vi "CALC_PAR_SEL.vi"(0 "VISA IN":refnum<visa-resource-name>, 1 "Measurement":string="CH1_S11_1", 5 "error in":errorcluster, 7 "Channel":i32=1) -> (14 "VISA Out":refnum<visa-resource-name>, 19 "error out":errorcluster)   [LabVIEW 2018, in "PNA-X.lvlib"]
doc: "CALCulate<cnum>:PARameter:SELect <Mname> \n1559\n\n(Read-Write) Sets the selected measurement. Most CALC: commands require that this command be \nsent before a setting change is made. One measurement on each channel can be selected at the same \ntime. To obtain a list of currently named measurements, use CALC:PAR:CAT? \nParameters \n<cnum> Channel number of the measurement to be selected. If unspecified, <cnum> is \nset to 1. \n<Mname> String - Name of the measurement. (Do NOT include the parameter name.) \nExamples CALC:PAR:SEL 'TEST' \ncalculate2:parameter:select 'test' \nQuery Syntax CALCulate:PARameter:SELect? \nReturn Type String \nDefault The preset measurement name is \"CH1_S11_1\" \nLast modified: \nApril 19, 2007 MX Added ADC meas \n9/12/06 MQ New Extended commands. \n1560\n\nCalculate:RData? Command \nCritical Note: CALCulate commands act on the selected measurement. You can select one \nmeasurement for each channel using Calc:Par:Select"
uses:
  PNA-X.lvlib
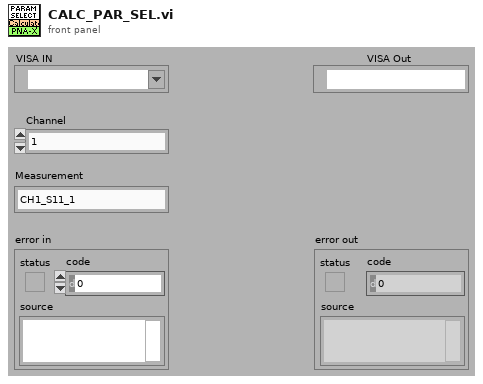
[diagram p1: front panel]
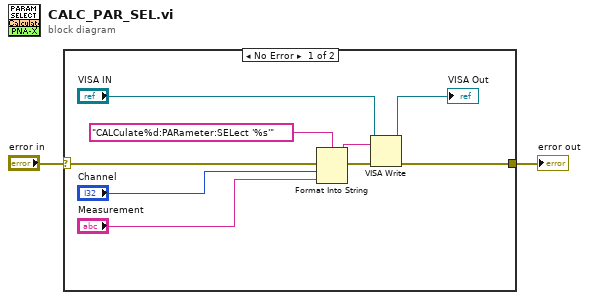
[diagram p0: block diagram]
diagram:
  n1 = case shown="No Error" "error in" {
    selector: "error in" -> [w11 w12]
    tunnel: [w6 w12] -> w1
    frame No Error {
      n2 = Format Into String(format string="CALCulate%d:PARameter:SELect '%s'" ("Cmdline"), error in=w11, "Channel", "Measurement") -> (resulting string=w9:string, error out=w10:errorcluster)  [unwired: 1 in]
      n3 = VISA Write(VISA resource name="VISA IN", write buffer=w9, error in (no error)=w10) -> (VISA resource name out=→"VISA Out":refnum<visa-resource-name>, error out=w6:errorcluster)  [unwired: 1 out]
    }
    frame Error {
    }
  }
  "error out" <- w1
